vi "Example 1.vi"() -> ()   [LabVIEW 2019]
uses:
  FINS/FINS_header.ctl
  FINS/FINS CMD.ctl
  subvi/task.ctl
  FINS/FINS TCP.lvlib
panel:
  out "data":bool[][](array[boolean])
  out "data":u8[](array[numeric])
  out "RSP":bool
  out "server Header":T1={"resp req"=FALSE, "cmd resp"=FALSE, "SID"=255, "DNA"=2, "DA1"=2, "DA2"=2, "SA1"=0, "SA2"=255, "SNA"=255} {"SNA" max=127 format="%x"; "SA2" max=254 step=1 format="%x"; "SA1" format="%x"; "DA2" max=254 step=1 format="%x"; "DA1" format="%x"; "DNA" max=127 step=1 format="%x"}
  out "server CMD":T2
  out "FINS Header":T1 {"SNA" max=127 format="%x"; "SA2" max=254 step=1 format="%x"; "SA1" format="%x"; "DA2" max=254 step=1 format="%x"; "DA1" format="%x"; "DNA" max=127 step=1 format="%x"}
  in  "SA1":u8 format="%x"
  out "Client Node":u32=10 format="%x"
  out "Server Node":u32=10 format="%x"
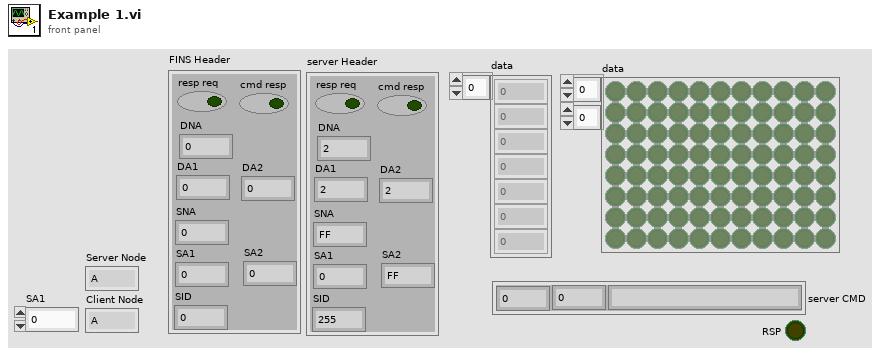
[diagram p1: front panel]
types:
  T1 = typedef "FINS TCP.lvlib/FINS_header.ctl" = cluster{"resp req":bool, "cmd resp":bool, "SID":u8, "DNA":u8, "DA1":u8, "DA2":u8, "SA1":u8, "SA2":u8, "SNA":u8}
  T2 = typedef "FINS TCP.lvlib/FINS CMD.ctl" = cluster{"MR":u8, "SR":u8, "name":string}
  T3 = typedef "task.ctl" = enum16{"connect", "send", "send-recv", "receive", "disconnect"}
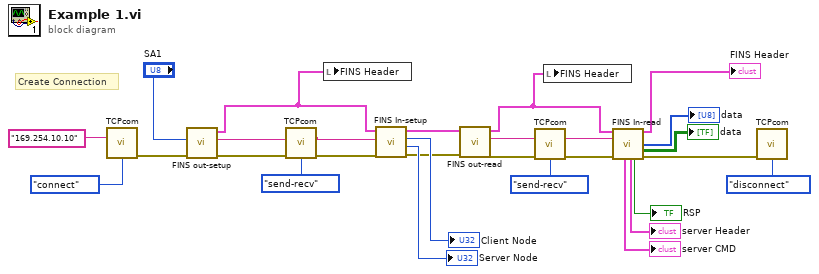
[diagram p0: block diagram]
diagram:
  # "Create Connection"
  n1 = call "TCPcom.vi"("string"="169.254.10.10" ("address"), "task"=task."connect") -> ("error out"=w27:errorcluster)  [unwired: 12 in, 1 out]
  n2 = call "FINS out-setup.vi"("error i"=w27, "SA1"="SA1") -> ("error o"=w25:errorcluster, "msg"=w26:string, "FINS Header"=w14:T1)  [unwired: 7 in]
  n3 = call "TCPcom.vi"("string"=w26, "error in"=w25, "task"=task."send-recv") -> ("data out"=w23:string, "error out"=w22:errorcluster)  [unwired: 11 in]
  n4 = local write "FINS Header"(w14) -> ()
  n5 = call "FINS In-setup.vi"("error i"=w22, "msg 3"=w23, "FINS Header i"=w14) -> ("error o"=w15:errorcluster, "Server Node"=→"Server Node":u32, "Client Node"=→"Client Node":u32, "FINS Header o"=w16:T1)  [unwired: 5 in]
  n6 = call "FINS out-read.vi"("error i"=w15, "FINS Header 2"=w16) -> ("error o"=w12:errorcluster, "msg"=w13:string, "FINS Header"=w3:T1)  [unwired: 7 in]
  n7 = call "TCPcom.vi"("string"=w13, "error in"=w12, "task"=task."send-recv") -> ("data out"=w11:string, "error out"=w10:errorcluster)  [unwired: 11 in]
  n8 = local write "FINS Header"(w3) -> ()
  n9 = call "FINS In-read.vi"("FINS Header i"=w3, "msg 3"=w11, "error i"=w10) -> ("FINS Header o"=→"FINS Header":T1, 8:"data"=→"data":u8[], 10:"data"=→"data":bool[][], "CMD"=→"server CMD":T2, "FINS Header 2"=→"server Header":T1, "RSP"=→"RSP":bool, "error o"=w5:errorcluster)  [unwired: 6 in]
  n10 = call "TCPcom.vi"("error in"=w5, "task"=task."disconnect") -> ()  [unwired: 12 in, 2 out]
